vi "Orca camera startup.vi"() -> ()   [LabVIEW 2011]
doc: "Cools down the camera to operating temperature before use and returns it to ambient after use. Run this VI before running any other ixon programs and leave it running the whole time you use the camera. To start: run vi, set temperature, check \"cooling\". To finish: Click \"warm up CCD and turn off camera\". Leave running until the program tells you that it has turned off the camera."
uses:
  Camera/camera globals.vi
panel:
  in  "Turn Off Camera":bool
  out "Status":string
  in  "error in (no error)":errorcluster
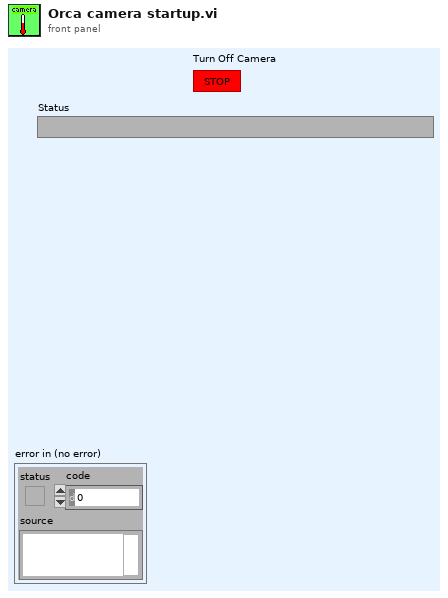
[diagram p1: front panel]
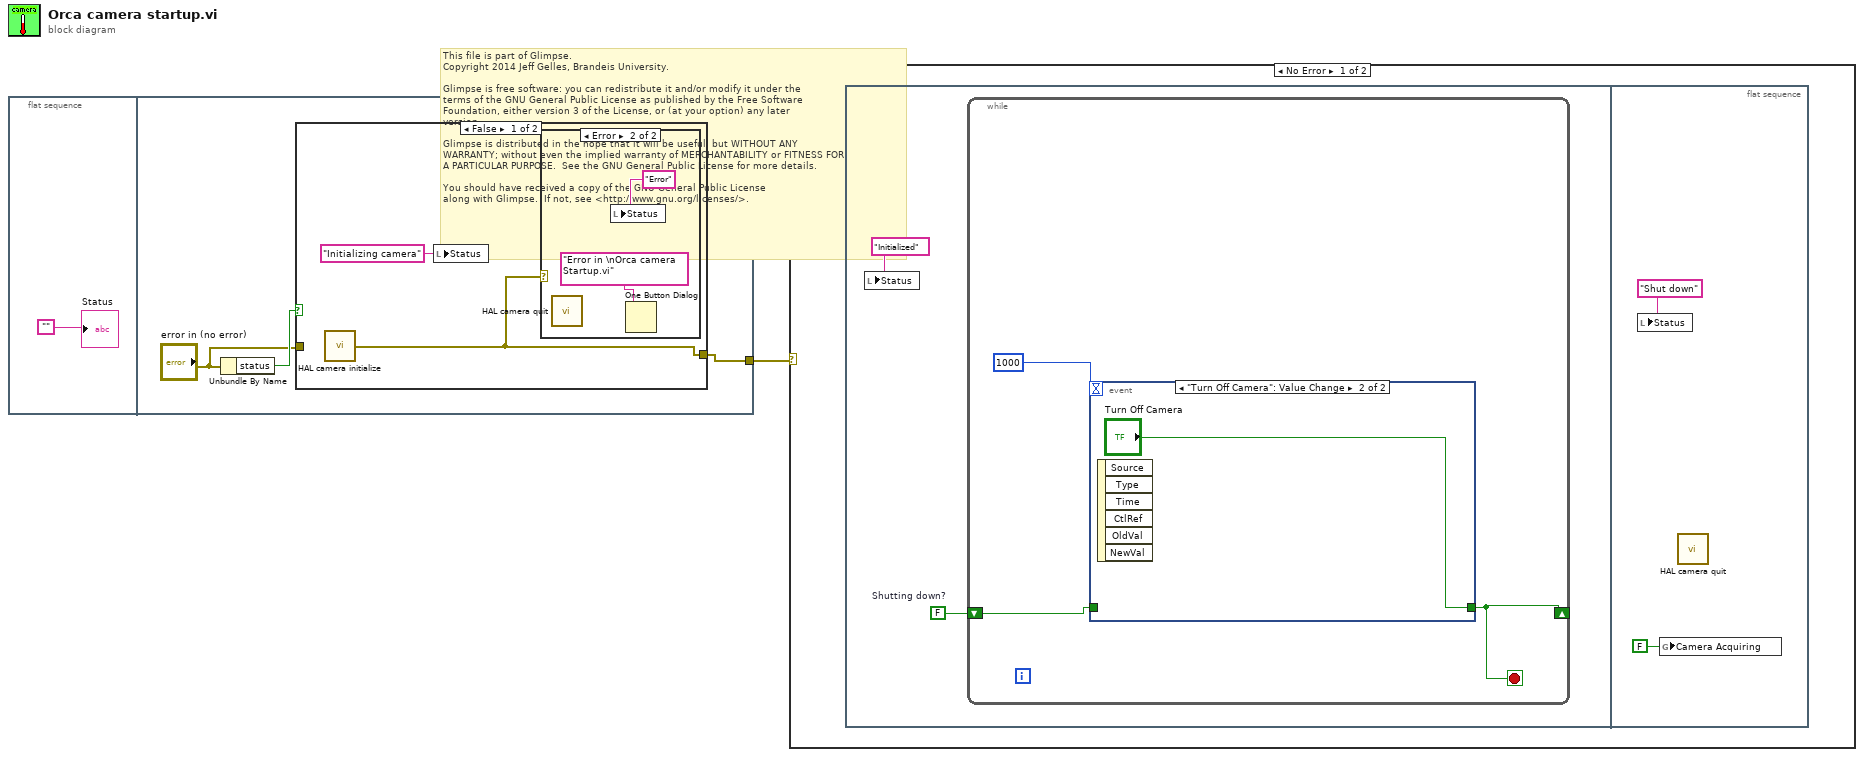
[diagram p0: block diagram]
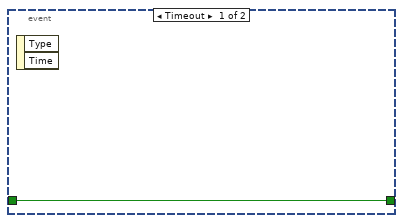
[diagram p2: hidden frame]
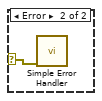
[diagram p3: hidden frame]
diagram:
  # "This file is part of Glimpse. \nCopyright 2014 Jeff Gelles, Brandeis University.    \n\nGlimpse is free software: you can redistribute it and/or modify it under the \nterms of the GNU General Public License as published by the Free Software \nFoundation, either version 3 of the License, or (at your option) any later \nversion.\n\nGlimpse is distributed in the hope that it will be useful, but WITHOUT ANY \nWARRANTY; without even the implied warranty of MERCHANTABILITY or FITNESS FOR \nA PARTICULAR PURPOSE.  See the GNU General Public License for more details.\n\nYou should have received a copy of the GNU General Public License\nalong with Glimpse.  If not, see <http://www.gnu.org/licenses/>."
  n1 = flat-sequence {
    tunnel: [w3] -> w1
    frame #0 {
      "Status" <- ""
    }
    frame #1 {
      n2 = Unbundle By Name("error in (no error)") -> ("status"=w5:bool)
      n3 = case shown="False" w5 {
        tunnel: [w6 w10] -> w3
        tunnel: "error in (no error)" -> [_ w10]
        frame False {
          n4 = call "HAL camera initialize.vi"() -> ("error out"=w6:errorcluster)
          n5 = local write "Status"("Initializing camera" ("Status")) -> ()
          n6 = case shown="Error" w6 {
            frame No Error {
            }
            frame Error {
              n7 = call "HAL camera quit.vi"() -> ()  [unwired: 1 out]
              n8 = local write "Status"("Error" ("Status")) -> ()
              n9 = One Button Dialog(message="Error in \nOrca camera Startup.vi" ("string")) -> ()  [unwired: 2 out]
            }
          }
        }
        frame True {
        }
      }
    }
  }
  n10 = case shown="No Error" w1 {
    selector: w1 -> [_ w20]
    frame No Error {
      n11 = flat-sequence {
        frame #0 {
          w12 = FALSE  # Shutting down?
          n12 = local write "Status"("Initialized" ("Status")) -> ()
          n13 = while {
            shift-right: [w13] -> _
            shift-left: w12 -> [w14]
            stop <- w13 stop-if-true
            n14 = event shown="[1] \"Turn Off Camera\": Value Change" {
              selector: _ -> [_ _]
              dyn-events: _ -> [_ _]
              timeout: 1000 -> [_ _]
              tunnel: w14 -> [w16 _]
              tunnel: [w16 "Turn Off Camera"] -> w13
              event Timeout {
                n15 = event-data() -> ()  [unwired: 3 out]
              }
              event "Turn Off Camera": Value Change {
                n16 = event-data() -> ()  [unwired: 7 out]
              }
            }
          }
        }
        frame #1 {
          n17 = local write "Status"("Shut down" ("Status")) -> ()
          n18 = global write "camera globals.vi" "Camera Acquiring"(FALSE ("Camera Acquiring")) -> ()
          n19 = call "HAL camera quit.vi"() -> ()  [unwired: 1 out]
        }
      }
    }
    frame Error {
      n20 = call <vilib>:"Simple Error Handler.vi"("error in (no error)"=w20) -> ()  [unwired: 1 in, 8 out]
    }
  }
